vi "treat request.vi"(8 "error in (no error)":errorcluster, 11 "S4GEI in":refnum<class "S4GEI.lvclass">) -> (0 "error out":errorcluster, 3 "S4GEI out":refnum<class "S4GEI.lvclass">)   [LabVIEW 2018, in "S4GEI.lvclass"]
uses:
  S4GEI.lvclass
  S4GEI.lvclass/S4GEI.ctl
  Channel GUI/Channel.lvclass/Channel.ctl
  State Machine/State Machine.lvclass
  Channel GUI/Channel.lvclass
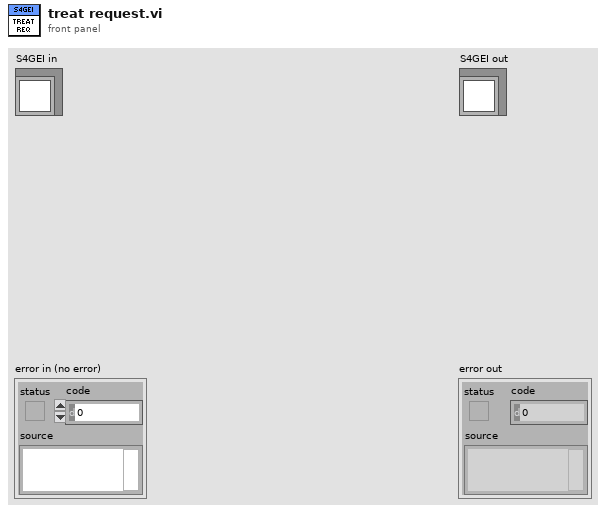
[diagram p1: front panel]
types:
  T1 = cluster{"State Machine.lvclass":refnum<class "State Machine.lvclass">, "RxTx.lvclass":refnum<class "RxTx.lvclass">, "Camera.lvclass":refnum<class "Camera.lvclass">, "Status RxTx.lvclass":refnum<class "RxTx.lvclass">}
  T2 = cluster{"frames":bool, "seqs":bool, "cycles":bool}
  T3 = cluster{"Acquire":bool, "Stop Acquisition":bool, "Abort Acquisition":bool, "Pause acquisition":bool}
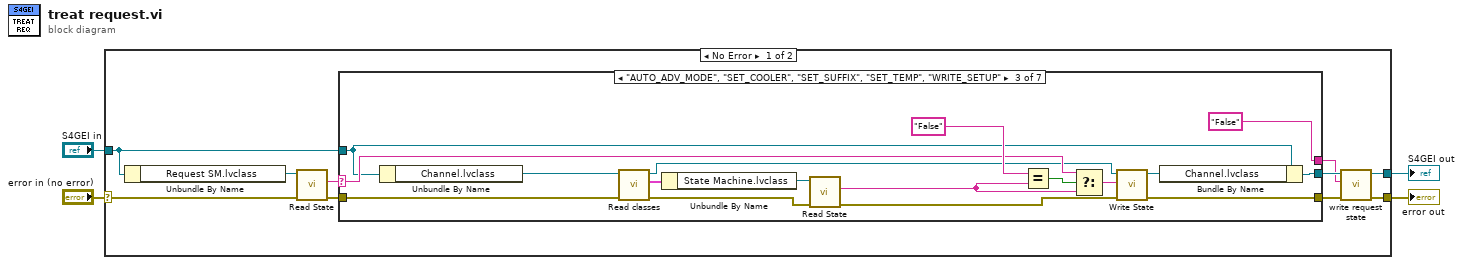
[diagram p0: block diagram]
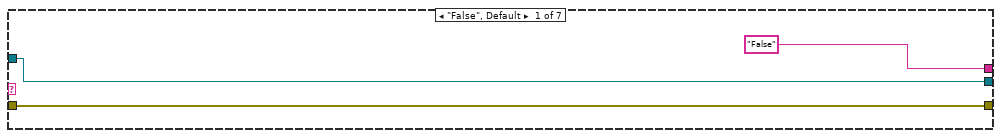
[diagram p2: hidden frame]
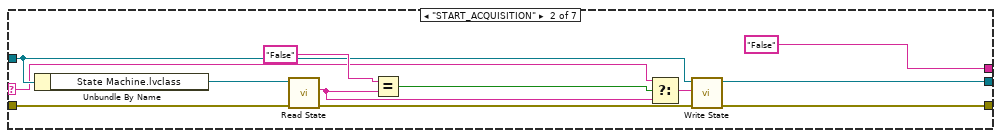
[diagram p3: hidden frame]
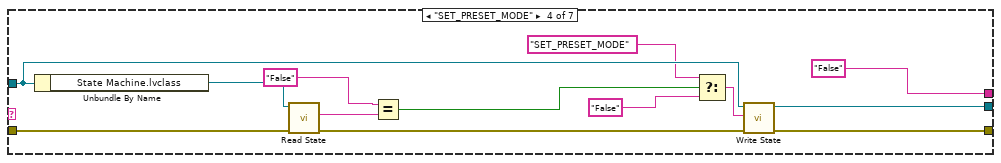
[diagram p4: hidden frame]
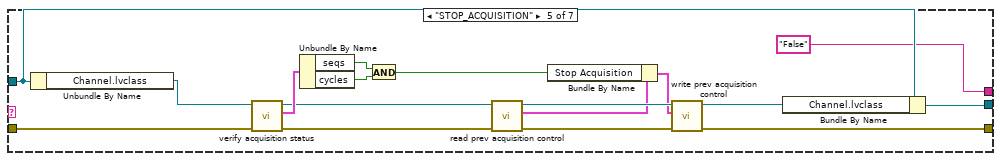
[diagram p5: hidden frame]
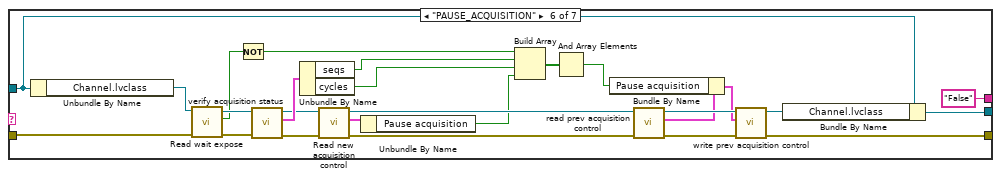
[diagram p6: hidden frame]
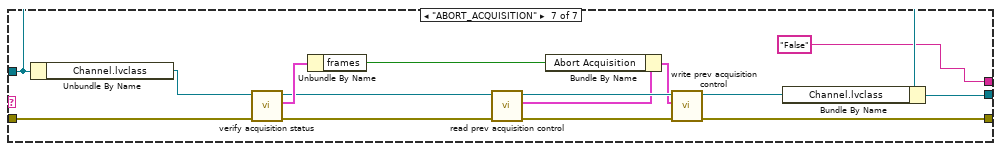
[diagram p7: hidden frame]
diagram:
  n1 = case shown="No Error" "error in (no error)" {
    selector: "error in (no error)" -> [w13 w119]
    tunnel: [w9 w119] -> w3
    tunnel: [w8 w118] -> w1
    tunnel: "S4GEI in" -> [w10 w118]
    frame No Error {
      n2 = Unbundle By Name(w10) -> ("Request SM.lvclass"=w14:refnum<class "State Machine.lvclass">)
      n3 = call-dynamic "Read State.vi"("error in (no error)"=w13, "State Machine in"=w14) -> ("error out"=w12:errorcluster, "State"=w11:string)  [unwired: 7 in, 1 out]
      n4 = case shown="\"AUTO_ADV_MODE\", \"SET_COOLER\", \"SET_SUFFIX\", \"SET_TEMP\", \"WRITE_SETUP\"" w11 {
        selector: w11 -> [_ w19 w43 _ _ _ _]
        tunnel: w12 -> [w17 w28 w41 w57 w75 w86 w116]
        tunnel: w10 -> [w16 w25 w33 w54 w63 w96 w107]
        tunnel: [w17 w22 w31 w47 w64 w97 w108] -> w6
        tunnel: [w16 w21 w30 w48 w61 w94 w105] -> w7
        tunnel: ["False" ("x") "False" ("x") "False" ("x") "False" ("x") "False" ("x") "False" ("x") "False" ("x")] -> w5
        frame "False", Default {
        }
        frame "START_ACQUISITION" {
          n5 = Unbundle By Name(w25) -> ("State Machine.lvclass"=w29:refnum<class "State Machine.lvclass">)
          n6 = call-dynamic "Read State.vi"("error in (no error)"=w28, "State Machine in"=w29) -> ("error out"=w26:errorcluster, "State"=w18:string)  [unwired: 7 in, 1 out]
          n7 = Equal?(x="False", y=w18) -> (x = y?=w24:bool)
          n8 = Select(t=w19, s=w24, f=w18) -> (s? t:f=w23:string)
          n9 = call "Write State.vi"("error in (no error)"=w26, "State"=w23, "SPARC4_GEI in"=w25) -> ("error out"=w22:errorcluster, "SPARC4_GEI out"=w21:refnum<class "S4GEI.lvclass">)  [unwired: 7 in]
        }
        frame "AUTO_ADV_MODE", "SET_COOLER", "SET_SUFFIX", "SET_TEMP", "WRITE_SETUP" {
          n10 = Unbundle By Name(w33) -> ("Channel.lvclass"=w42:refnum<class "Channel.lvclass">)
          n11 = call-dynamic "Read classes.vi"("error in (no error)"=w41, "Channel in"=w42) -> ("error out"=w38:errorcluster, "classes"=w40:T1, "Channel out"=w36:refnum<class "Channel.lvclass">)  [unwired: 7 in]
          n12 = Unbundle By Name(w40) -> ("State Machine.lvclass"=w39:refnum<class "State Machine.lvclass">)
          n13 = call-dynamic "Read State.vi"("error in (no error)"=w38, "State Machine in"=w39) -> ("error out"=w35:errorcluster, "State"=w37:string)  [unwired: 7 in, 1 out]
          n14 = Equal?(x="False", y=w37) -> (x = y?=w45:bool)
          n15 = Select(t=w43, s=w45, f=w37) -> (s? t:f=w34:string)
          n16 = call "Write State.vi"("error in (no error)"=w35, "State"=w34, "Channel GEI in"=w36) -> ("error out"=w31:errorcluster, "Channel GEI out"=w32:refnum<class "Channel.lvclass">)  [unwired: 7 in]
          n17 = Bundle By Name(cluster=w33, "Channel.lvclass"=w32) -> (w30:refnum<class "S4GEI.lvclass">)
        }
        frame "SET_PRESET_MODE" {
          n18 = Unbundle By Name(w54) -> ("State Machine.lvclass"=w58:refnum<class "State Machine.lvclass">)
          n19 = call-dynamic "Read State.vi"("error in (no error)"=w57, "State Machine in"=w58) -> ("error out"=w53:errorcluster, "State"=w56:string)  [unwired: 7 in, 1 out]
          n20 = Equal?(x="False", y=w56) -> (x = y?=w52:bool)
          n21 = Select(t="SET_PRESET_MODE", s=w52, f="False") -> (s? t:f=w49:string)
          n22 = call "Write State.vi"("error in (no error)"=w53, "State"=w49, "SPARC4_GEI in"=w54) -> ("error out"=w47:errorcluster, "SPARC4_GEI out"=w48:refnum<class "S4GEI.lvclass">)  [unwired: 7 in]
        }
        frame "STOP_ACQUISITION" {
          n23 = Unbundle By Name(w63) -> ("Channel.lvclass"=w76:refnum<class "Channel.lvclass">)
          n24 = call "verify acquisition status.vi"("error in (no error)"=w75, "Channel in"=w76) -> ("error out"=w71:errorcluster, "acq status"=w74:T2, "Channel out"=w68:refnum<class "Channel.lvclass">)  [unwired: 7 in]
          n25 = Unbundle By Name(w74) -> ("seqs"=w73:bool, "cycles"=w72:bool)
          n26 = And(x=w73, y=w72) -> (x .and. y?=w65:bool)
          n27 = call-dynamic "read prev acquisition control.vi"("error in (no error)"=w71, "Channel in"=w68) -> ("error out"=w69:errorcluster, "prev acquisition control"=w67:T3, "Channel out"=w70:refnum<class "Channel.lvclass">)  [unwired: 7 in]
          n28 = Bundle By Name(cluster=w67, "Stop Acquisition"=w65) -> (w66:T3)
          n29 = call-dynamic "write prev acquisition control.vi"("error in (no error)"=w69, "prev acquisition control"=w66, "Channel in"=w70) -> ("error out"=w64:errorcluster, "Channel out"=w62:refnum<class "Channel.lvclass">)  [unwired: 7 in]
          n30 = Bundle By Name(cluster=w63, "Channel.lvclass"=w62) -> (w61:refnum<class "S4GEI.lvclass">)
        }
        frame "PAUSE_ACQUISITION" {
          n31 = Unbundle By Name(w96) -> ("Channel.lvclass"=w87:refnum<class "Channel.lvclass">)
          n32 = call-dynamic "Read wait expose.vi"("error in (no error)"=w86, "Channel in"=w87) -> ("error out"=w85:errorcluster, "wait expose"=w77:bool, "Channel out"=w84:refnum<class "Channel.lvclass">)  [unwired: 7 in]
          n33 = Not(x=w77) -> (.not. x?=w78:bool)
          n34 = call "verify acquisition status.vi"("error in (no error)"=w85, "Channel in"=w84) -> ("error out"=w91:errorcluster, "acq status"=w102:T2, "Channel out"=w92:refnum<class "Channel.lvclass">)  [unwired: 7 in]
          n35 = Unbundle By Name(w102) -> ("seqs"=w83:bool, "cycles"=w82:bool)
          n36 = call "Read new acquisition control.vi"("error in (no error)"=w91, "Channel in"=w92) -> ("error out"=w90:errorcluster, "new acquisition control"=w88:T3, "Channel out"=w89:refnum<class "Channel.lvclass">)  [unwired: 7 in]
          n37 = Unbundle By Name(w88) -> ("Pause acquisition"=w81:bool)
          n38 = Build Array(w78, w83, w82, w81) -> (w80:bool[])
          n39 = And Array Elements(Boolean array=w80) -> (logical AND=w79:bool)
          n40 = call-dynamic "read prev acquisition control.vi"("error in (no error)"=w90, "Channel in"=w89) -> ("error out"=w100:errorcluster, "prev acquisition control"=w99:T3, "Channel out"=w101:refnum<class "Channel.lvclass">)  [unwired: 7 in]
          n41 = Bundle By Name(cluster=w99, "Pause acquisition"=w79) -> (w98:T3)
          n42 = call-dynamic "write prev acquisition control.vi"("error in (no error)"=w100, "prev acquisition control"=w98, "Channel in"=w101) -> ("error out"=w97:errorcluster, "Channel out"=w95:refnum<class "Channel.lvclass">)  [unwired: 7 in]
          n43 = Bundle By Name(cluster=w96, "Channel.lvclass"=w95) -> (w94:refnum<class "S4GEI.lvclass">)
        }
        frame "ABORT_ACQUISITION" {
          n44 = Unbundle By Name(w107) -> ("Channel.lvclass"=w117:refnum<class "Channel.lvclass">)
          n45 = call "verify acquisition status.vi"("error in (no error)"=w116, "Channel in"=w117) -> ("error out"=w114:errorcluster, "acq status"=w115:T2, "Channel out"=w111:refnum<class "Channel.lvclass">)  [unwired: 7 in]
          n46 = Unbundle By Name(w115) -> ("frames"=w103:bool)
          n47 = call-dynamic "read prev acquisition control.vi"("error in (no error)"=w114, "Channel in"=w111) -> ("error out"=w112:errorcluster, "prev acquisition control"=w110:T3, "Channel out"=w113:refnum<class "Channel.lvclass">)  [unwired: 7 in]
          n48 = Bundle By Name(cluster=w110, "Abort Acquisition"=w103) -> (w109:T3)
          n49 = call-dynamic "write prev acquisition control.vi"("error in (no error)"=w112, "prev acquisition control"=w109, "Channel in"=w113) -> ("error out"=w108:errorcluster, "Channel out"=w106:refnum<class "Channel.lvclass">)  [unwired: 7 in]
          n50 = Bundle By Name(cluster=w107, "Channel.lvclass"=w106) -> (w105:refnum<class "S4GEI.lvclass">)
        }
      }
      n51 = call "write request state.vi"("error in (no error)"=w6, "State"=w5, "S4GEI in"=w7) -> ("error out"=w9:errorcluster, "S4GEI out"=w8:refnum<class "S4GEI.lvclass">)  [unwired: 7 in]
    }
    frame Error {
    }
  }
  "error out" <- w3
  "S4GEI out" <- w1
